vi "ErrorHelper.vi"(1 "Message":string, 2 "Code":i32, 3 "This VI":refnum<vi>) -> (0 "error out":errorcluster)   [LabVIEW 2011, in "Konvolucio MUDS150628.lvlib"]
uses:
  <instrlib>/Konvolucio MUDS150628/Konvolucio MUDS150628.lvlib
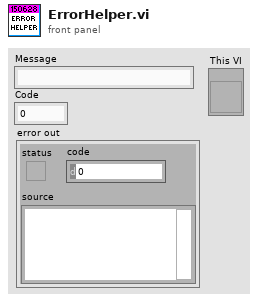
[diagram p1: front panel]
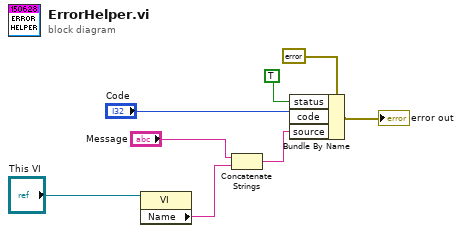
[diagram p0: block diagram]
diagram:
  n1 = property class="VI"(reference="This VI") -> ("Name"=w1:string)  [unwired: 1 in, 2 out]
  n2 = Concatenate Strings("Message", w1) -> (w7:string)
  n3 = Bundle By Name(cluster=errorcluster {"status"=FALSE, "code"=0, "source"=""} ("error out"), "status"=TRUE, "code"="Code", "source"=w7) -> (→"error out":errorcluster)
